vi "Calculate Port.vi"(8 "error in (no error)":errorcluster, 11 "TCP Server in":refnum<class "TCP Server.lvclass">) -> (0 "error out":errorcluster, 2 "Port":u16, 3 "TCP Server out":refnum<class "TCP Server.lvclass">)   [LabVIEW 2026, in "TALOS.lvlib" / "TCP Server.lvlib" / "TCP Server.lvclass"]
uses:
  TCP Server.lvclass
  C:/LabVIEW Code/TALOS/talos/Ancestor/Ancestor/Ancestor.lvclass
  Ancestor/Ancestor/Ancestor.lvclass/Ancestor.ctl
  Ancestor/Ancestor/Read ID.vi
  TALOS.lvlib
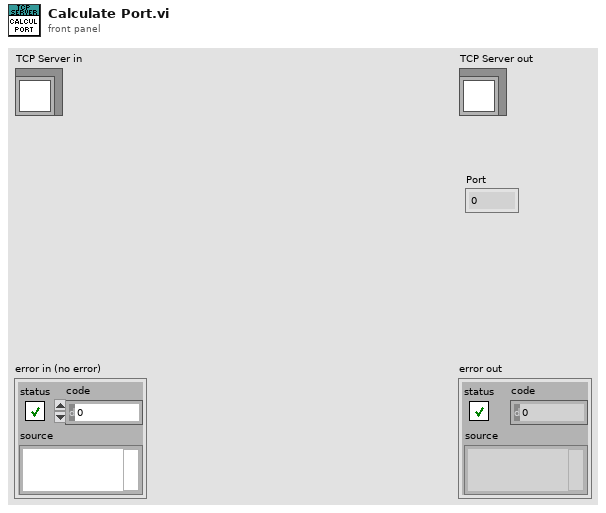
[diagram p1: front panel]
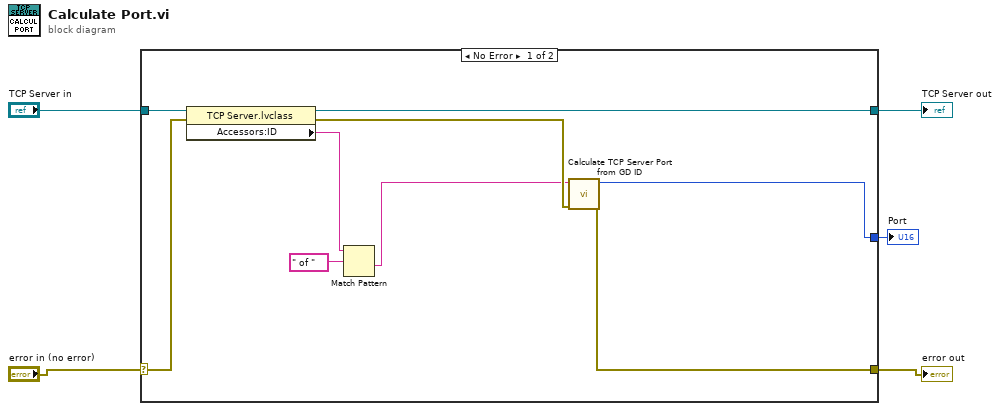
[diagram p0: block diagram]
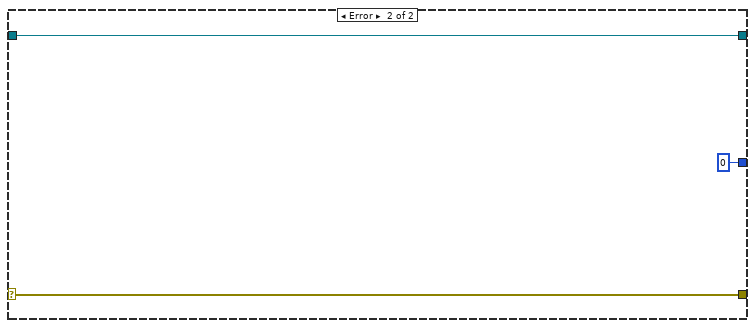
[diagram p2: hidden frame]
diagram:
  n1 = case shown="No Error" "error in (no error)" {
    selector: "error in (no error)" -> [w12 w15]
    tunnel: [w11 w17] -> w4
    tunnel: "TCP Server in" -> [w10 w17]
    tunnel: [w7 u16 0] -> w3
    tunnel: [w14 w15] -> w1
    frame No Error {
      n2 = property class="TCP Server.lvclass"(reference=w10, error in=w12) -> (reference out=w11:refnum<class "TCP Server.lvclass">, error out=w13:errorcluster, "Accessors:ID"=w9:string)
      n3 = Match Pattern(string=w9, regular expression=" of " ("string")) -> (after substring=w6:string)  [unwired: 1 in, 3 out]
      n4 = call "Calculate TCP Server Port from GD ID.vi"("error in (no error)"=w13, "GD ID"=w6) -> ("error out"=w14:errorcluster, "Port"=w7:u16)  [unwired: 8 in]
    }
    frame Error {
    }
  }
  "error out" <- w1
  "TCP Server out" <- w4
  "Port" <- w3
